vi "3DplotterDataStore.vi"(10 "3DplotterDataIn":T1 {"vector2Info"."UVW-TI" format="%#_3g"; "vector2Info"."XYZ-WD" format="%#_3g"; "vector1Info"."UVW-TI" format="%#_3g"; "vector1Info"."XYZ-WD" format="%#_3g"}) -> (2 "3DplotterDataOut":T1 {"vector2Info"."UVW-TI" format="%#_3g"; "vector2Info"."XYZ-WD" format="%#_3g"; "vector1Info"."UVW-TI" format="%#_3g"; "vector1Info"."XYZ-WD" format="%#_3g"})   [LabVIEW 2021]
uses:
  3DplotterData.ctl
  vectorDef.ctl
panel:
  # "Avoids the need for train tracks on calling VI, and provides visibility for data cluster"
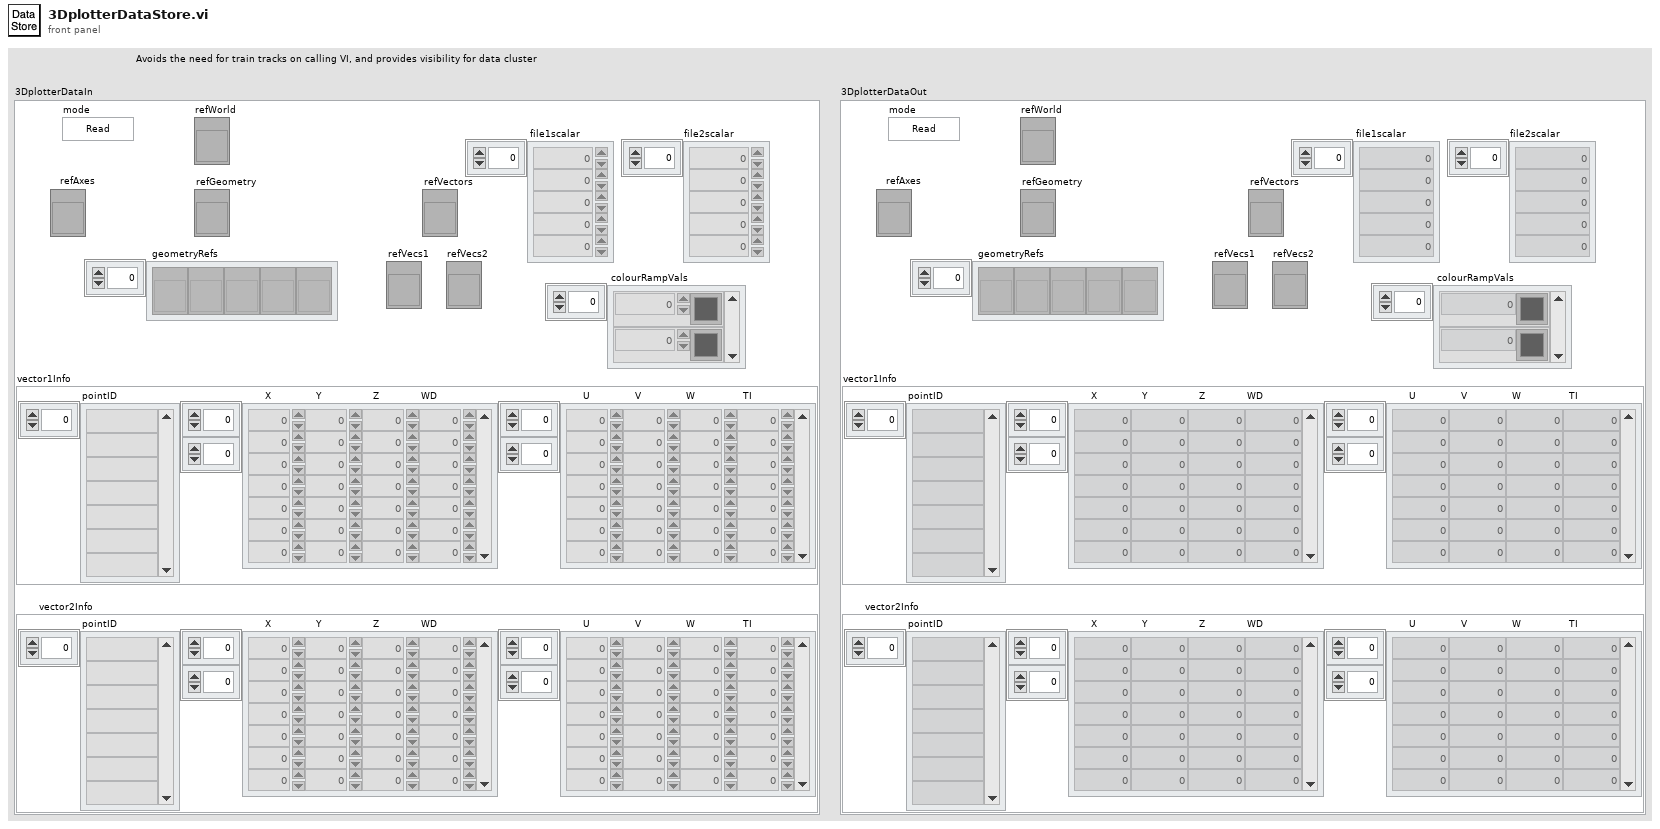
[diagram p1: front panel]
types:
  T1 = typedef "3DplotterData.ctl" = cluster{"mode":bool, "refWorld":refnum<vi>, "refAxes":refnum<vi>, "refVectors":refnum<vi>, "refVecs1":refnum<vi>, "refVecs2":refnum<vi>, "vector1Info":T2, "file1scalar":dbl[], "vector2Info":T2, "file2scalar":dbl[], "colourRampVals":cluster{"value":dbl, "colour":u32}[], "geometryRefs":refnum<vi>[], "refGeometry":refnum<vi>}
  T2 = typedef "vectorDef.ctl" = cluster{"pointID":string[], "XYZ-WD":dbl[][], "UVW-TI":dbl[][]}
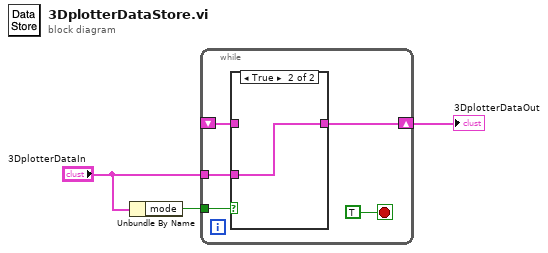
[diagram p0: block diagram]
diagram:
  n1 = Unbundle By Name("3DplotterDataIn") -> ("mode"=w1:bool)
  n2 = while {
    shift-right: [w8] -> w3
    shift-left: _ -> [w6]
    tunnel: "3DplotterDataIn" -> [w7]
    tunnel: w1 -> [w4]
    stop <- TRUE stop-if-true
    n3 = case shown="True" w4 {
      tunnel: [w9 w10] -> w8
      tunnel: w7 -> [_ w10]
      tunnel: w6 -> [w9 _]
      frame False {
      }
      frame True {
      }
    }
  }
  "3DplotterDataOut" <- w3
